vi "Format Address List.vi"(10 "Addresses":T1[](array[typedef])) -> (2 "Address List":string)   [LabVIEW 2020, in "Gmail API.lvlib" / "Gmail.lvclass"]
uses:
  Gmail.lvclass
  Mail Address.ctl
  Gmail API.lvlib
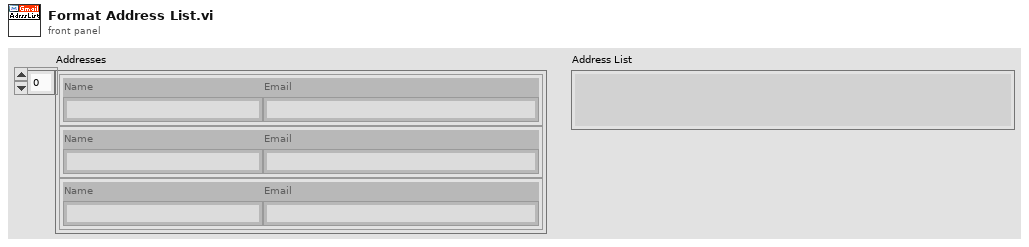
[diagram p1: front panel]
types:
  T1 = typedef "Gmail API.lvlib/Mail Address.ctl" = cluster{"Name":string, "Email":string}
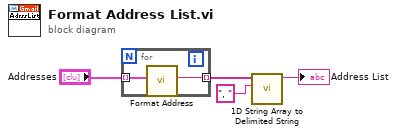
[diagram p0: block diagram]
diagram:
  n1 = for {
    tunnel: "Addresses" -> [w6] mode=indexing
    tunnel: [w5] -> w3 mode=indexing
    n2 = call "Format Address.vi"("Address"=w6) -> ("Formatted Address"=w5:string)  [unwired: 10 in]
  }
  n3 = call <vilib>:"1D String Array to Delimited String.vi"("delimiter"=", ", "string array"=w3) -> ("delimited string"=→"Address List":string)  [unwired: 9 in]
